vi "Join Strings.vi"(10 "구분자 (\", \")":string=", ", 11 "문자열":string[](array[string])) -> (3 "합쳐진 문자열":string)   [LabVIEW 2010]
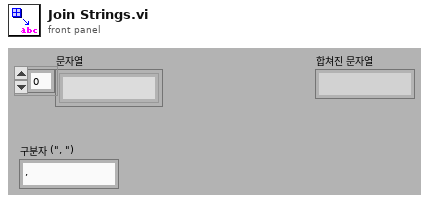
[diagram p1: front panel]
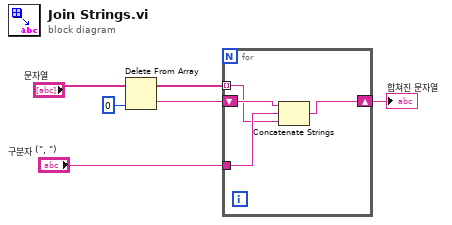
[diagram p0: block diagram]
diagram:
  n1 = Delete From Array(array="문자열", index=0) -> (deleted portion=w5:string, array with subset deleted=w3:string[])  [unwired: 1 in]
  n2 = for {
    shift-right: [w7] -> w2
    shift-left: w5 -> [w10]
    tunnel: "구분자 (\", \")" -> [w9]
    tunnel: w3 -> [w8] mode=indexing
    n3 = Concatenate Strings(w10, w9, w8) -> (w7:string)
  }
  "합쳐진 문자열" <- w2
